vi "getCurrentPath.vi"(8 "error in (no error)":errorcluster, 11 "SettingsManager.lvclass in":refnum<class "SettingsManager.lvclass">) -> (0 "error out":errorcluster, 2 "Current Path":path=path "D:/Data/Labview/BEC Suite/Hal/Channels/Camera/XML Camera Settings/CameraSettings.xml", 3 "SettingsManager.lvclass out":refnum<class "SettingsManager.lvclass">)   [LabVIEW 2011, in "Tools.lvlib" / "Settings.lvlib" / "SettingsManager.lvclass"]
uses:
  SettingsManager.lvclass
  SettingsManager.lvclass/SettingsManager.ctl
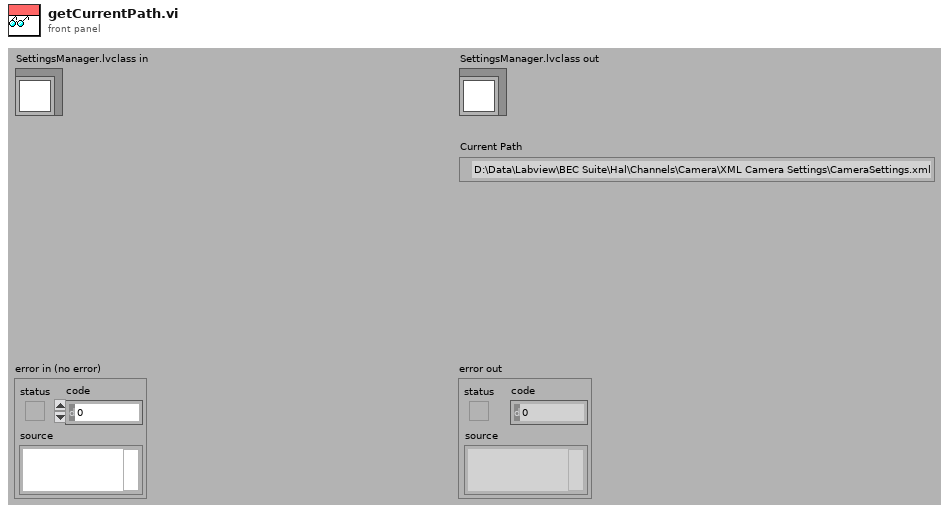
[diagram p1: front panel]
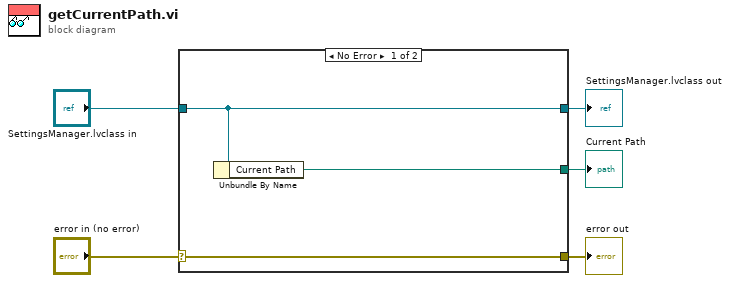
[diagram p0: block diagram]
diagram:
  n1 = case shown="No Error" "error in (no error)" {
    selector: "error in (no error)" -> [w8 w9]
    tunnel: [w8 w9] -> w4
    tunnel: [w7 w10] -> w2
    tunnel: "SettingsManager.lvclass in" -> [w7 w10]
    tunnel: [w6 _] -> w1
    frame No Error {
      n2 = Unbundle By Name(w7) -> ("Current Path"=w6:path)
    }
    frame Error {
    }
  }
  "error out" <- w4
  "SettingsManager.lvclass out" <- w2
  "Current Path" <- w1
